vi "CheckState.vi"(10 "Input":string) -> (2 "IP State":bool)   [LabVIEW 2020, in "Controller.lvlib"]
uses:
  Controller.lvlib
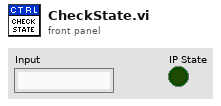
[diagram p1: front panel]
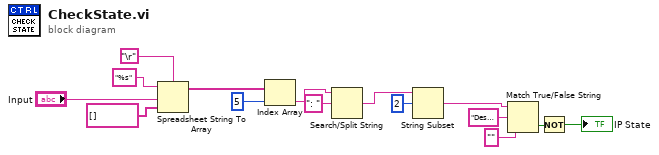
[diagram p0: block diagram]
diagram:
  n1 = Spreadsheet String To Array(delimiter (Tab)="\r", format string="%s", spreadsheet string="Input", array type (2D Dbl)=string[] []) -> (array=w12:string[])
  n2 = Index Array(array=w12, index=5) -> (element=w7:string)
  n3 = Search/Split String(string=w7, search string/char (-)=": ") -> (match + rest of string=w10:string)  [unwired: 1 in, 2 out]
  n4 = String Subset(string=w10, offset (0)=2) -> (substring=w4:string)  [unwired: 1 in]
  n5 = Match True/False String(2:"" ("false string"), 3:"Destination host unreachable." ("true string"), 4:w4) -> (0:w5:bool)  [unwired: 1 out]
  n6 = Not(x=w5) -> (.not. x?=→"IP State":bool)
